vi "Calc Rotation Value.vi"(2 "Gyro Angle":dbl, 3 "Joystick Rotation":dbl, 4 "Rotation Data":T1) -> (0 "Rotation Value":dbl)   [LabVIEW 2019]
uses:
  <vilib>/addons/control/pid/NI_PID_pid.lvlib
  <vilib>/Rock Robotics/Network Tables/NT Write Boolean.vi
  <vilib>/Rock Robotics/Network Tables/NT Write Number.vi
  <vilib>/addons/control/pid/pid.llb/PID (DBL).vi
  Controls/DriveJoystickData.ctl
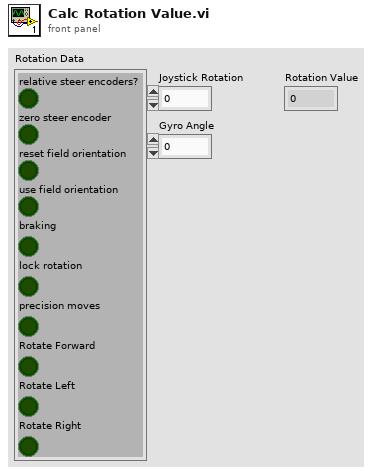
[diagram p1: front panel]
types:
  T1 = typedef "DriveJoystickData.ctl" = cluster{"relative steer encoders?":bool, "zero steer encoder":bool, "reset field orientation":bool, "use field orientation":bool, "braking":bool, "lock rotation":bool, "precision moves":bool, "Rotate Forward":bool, "Rotate Left":bool, "Rotate Right":bool}
  T2 = cluster{"proportional gain (Kc)":dbl, "integral time (Ti, min)":dbl, "derivative time (Td, min)":dbl}
  T3 = typedef "WPI_JoystickDevRef.ctl" = cluster{"Device":T4}
  T4 = typedef "WPI_JoystickDeviceEnum.ctl" = enum16{"USB 0", "USB 1", "USB 2", "USB 3", "USB 4", "USB 5"}
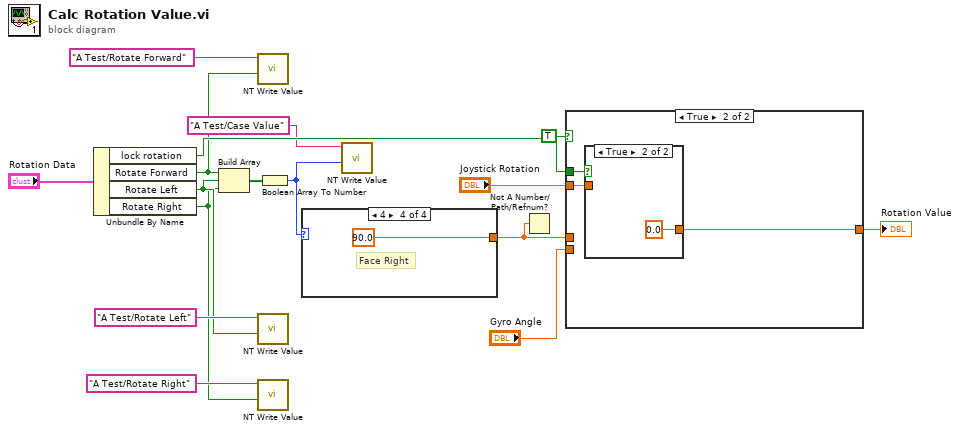
[diagram p0: block diagram]
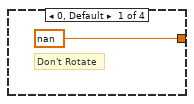
[diagram p2: hidden frame]
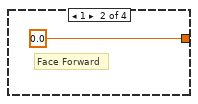
[diagram p3: hidden frame]
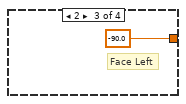
[diagram p4: hidden frame]
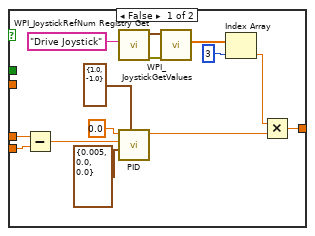
[diagram p5: hidden frame]
diagram:
  n1 = Unbundle By Name("Rotation Data") -> ("lock rotation"=w14:bool, "Rotate Forward"=w9:bool, "Rotate Left"=w6:bool, "Rotate Right"=w4:bool)
  n2 = Build Array(w9, w6, w4) -> (w12:bool[])
  n3 = call-poly <vilib>:"NT Write Value.vi"("Boolean"=w9, "Name"="A Test/Rotate Forward") -> ()  [unwired: 9 in, 1 out]
  n4 = call-poly <vilib>:"NT Write Value.vi"("Boolean"=w6, "Name"="A Test/Rotate Left") -> ()  [unwired: 9 in, 1 out]
  n5 = call-poly <vilib>:"NT Write Value.vi"("Boolean"=w4, "Name"="A Test/Rotate Right") -> ()  [unwired: 9 in, 1 out]
  n6 = Boolean Array To Number(Boolean array=w12) -> (number=w2:u32)
  n7 = case shown="4" w2 {
    tunnel: [nan 0.0 -90.0 90.0] -> w10
    frame 0, Default {
      # "Don't Rotate"
    }
    frame 1 {
      # "Face Forward"
    }
    frame 2 {
      # "Face Left"
    }
    frame 4 {
      # "Face Right"
    }
  }
  n8 = call-poly <vilib>:"NT Write Value.vi"("Numeric"=w2, "Name"="A Test/Case Value") -> ()  [unwired: 9 in, 1 out]
  n9 = Not A Number/Path/Refnum?(number/path/refnum=w10) -> ()  [unwired: 1 out]
  n10 = case shown="True" TRUE {
    tunnel: "Joystick Rotation" -> [_ w35]
    tunnel: w14 -> [_ w37]
    tunnel: [w28 w36] -> w13
    tunnel: "Gyro Angle" -> [w34 _]
    tunnel: w10 -> [w33 _]
    frame False {
      n11 = Subtract(x=w33, y=w34) -> (x-y=w32:dbl)
      n12 = call <vilib>:"WPI_JoystickRefNum Registry Get.vi"("refnum name"="Drive Joystick") -> ("error out"=w25:errorcluster, "JoystickDevRef"=w26:T3)  [unwired: 9 in]
      n13 = call-poly <vilib>:"PID.vi"("output range"=cluster{"output high":dbl, "output low":dbl} {"output high"=1.0, "output low"=-1.0}, "PID gains"=T2 {"proportional gain (Kc)"=0.005, "integral time (Ti, min)"=0.0, "derivative time (Td, min)"=0.0}, "process variable"=w32, "setpoint"=0.0) -> ("output"=w21:dbl)  [unwired: 6 in, 1 out]
      n14 = call <vilib>:"WPI_JoystickGetValues.vi"("error in (no error)"=w25, "JoystickDevRef"=w26) -> ("Axes"=w27:dbl[])  [unwired: 5 in, 4 out]
      n15 = Index Array(array=w27, index=3) -> (element=w22:dbl)
      n16 = Multiply(x=w22, y=w21) -> (x*y=w28:dbl)
    }
    frame True {
      n17 = case shown="True" w37 {
        tunnel: [w38 0.0] -> w36
        tunnel: w35 -> [w38 _]
        frame False {
        }
        frame True {
        }
      }
    }
  }
  "Rotation Value" <- w13
